vi "四通道数据采集.vi"() -> ()   [LabVIEW 2012, in "Mlistbox Tools.lvlib"]
uses:
  Mlistbox Tools.lvlib
  ListBox/Custom Type/Read and Write Mode.ctl
  Method/Clear.vi
  Property/Set and Get Row or Col Head Strings.vi
  Method/Add Item.vi
  Method/Add Item Buffered.vi
  Method/Sort.vi
  ListBox/Listbox Tool.lvlib
panel:
  out "Selected Item":string[](array[string])
  in  "清除项目":bool
  in  "缓冲添加项目":bool
  in  "停止按钮":bool
  in  "多列列表框":i32(listbox)
  # "双击列首自动排序"
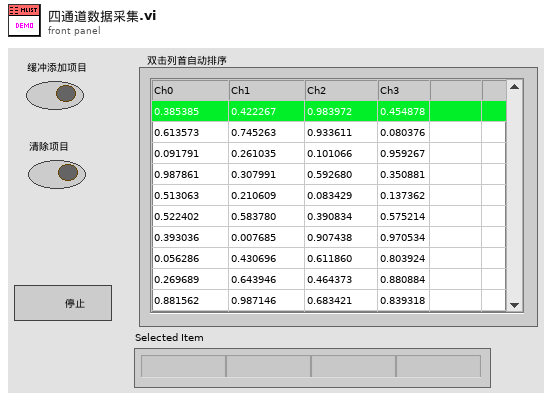
[diagram p1: front panel]
types:
  T1 = typedef "Listbox Tool.lvlib/Read and Write Mode.ctl" = enum16{"Read", "Write"}
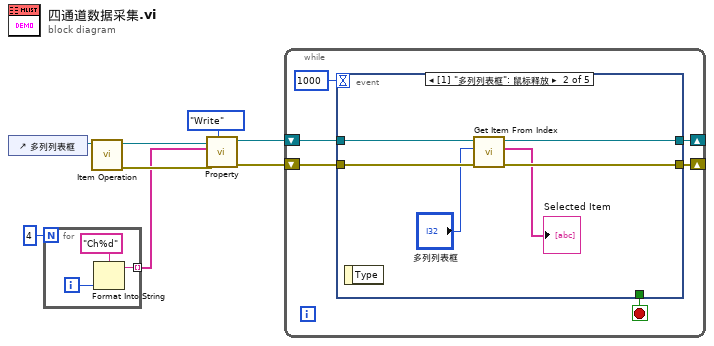
[diagram p0: block diagram]
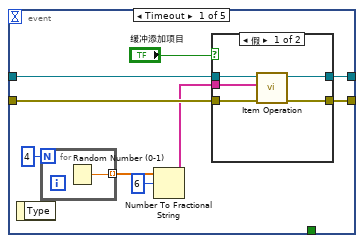
[diagram p2: hidden frame]
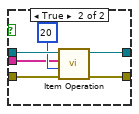
[diagram p3: hidden frame]
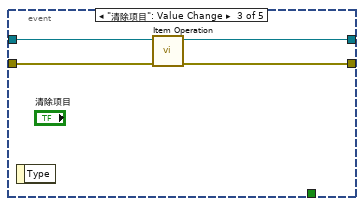
[diagram p4: hidden frame]
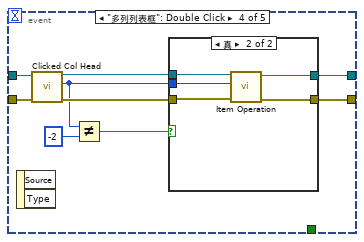
[diagram p5: hidden frame]
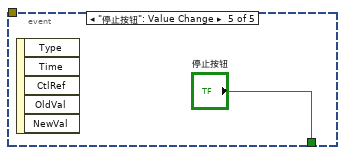
[diagram p7: hidden frame]
diagram:
  n1 = control-ref of="多列列表框"() -> (w8:refnum<vi>)
  n2 = for {
    N: 4 -> [_]
    tunnel: [w9] -> w4 mode=indexing
    i -> [w11]
    n3 = Format Into String(format string="Ch%d" ("格式字符串"), w11) -> (resulting string=w9:string)  [unwired: 2 in, 1 out]
  }
  n4 = call-poly "Item Operation.vi"("Mlistbox Ref"=w8) -> ("错误输出"=w6:errorcluster, "Mlistbox Ref Dup"=w7:refnum<vi>)  [unwired: 9 in]
  n5 = call-poly "Property.vi"("Mode"=Read_and_Write_Mode."Write", "错误输入"=w6, "String[]  In"=w4, "Mlistbox Ref"=w7) -> ("错误输出"=w1:errorcluster, "Mlistbox Ref Dup"=w2:refnum<vi>)  [unwired: 5 in, 1 out]
  n6 = while {
    shift-right: [w14] -> _
    shift-left: w2 -> [w15]
    shift-right: [w13] -> _
    shift-left: w1 -> [w16]
    stop <- w17 stop-if-true
    n7 = event shown="[1] \"多列列表框\": 鼠标释放" {
      selector: _ -> [_ _ _ _ _]
      dyn-events: _ -> [_ _ _ _ _]
      timeout: 1000 -> [_ _ _ _ _]
      tunnel: [_ _ _ _ "停止按钮"] -> w17
      tunnel: w16 -> [w26 w43 w47 w55 _]
      tunnel: w15 -> [w25 w44 w48 w54 _]
      tunnel: [w24 w41 w45 w57 _] -> w14
      tunnel: [w23 w42 w46 w56 _] -> w13
      event Timeout {
        n8 = event-data() -> ()  [unwired: 1 in, 1 out]
        n9 = for {
          N: 4 -> [_]
          tunnel: [w38] -> w21 mode=indexing
          n10 = Random Number (0-1)() -> (number: 0 to 1=w38:dbl)
        }
        n11 = Number To Fractional String(number=w21, width (-)=i16 6 ("宽度(-)")) -> (F-format string=w20:string[])  [unwired: 2 in]
        n12 = case shown="假" "缓冲添加项目" {
          tunnel: w26 -> [w31 w37]
          tunnel: w25 -> [w28 w36]
          tunnel: [w29 w35] -> w24
          tunnel: [w30 w34] -> w23
          tunnel: w20 -> [w27 w32]
          frame False {
            n13 = call-poly "Item Operation.vi"("错误输入"=w31, "Item"=w27, "Mlistbox Ref"=w28) -> ("错误输出"=w30:errorcluster, "Mlistbox Ref Dup"=w29:refnum<vi>)  [unwired: 7 in]
          }
          frame True {
            n14 = call-poly "Item Operation.vi"("错误输入"=w37, "Length"=20, "Item"=w32, "Mlistbox Ref"=w36) -> ("错误输出"=w34:errorcluster, "Mlistbox Ref Dup"=w35:refnum<vi>)  [unwired: 6 in]
          }
        }
      }
      event "多列列表框": Mouse Up {
        n15 = event-data() -> ()  [unwired: 1 in, 1 out]
        n16 = call "Get Item From Index.vi"("错误输入"=w43, "Index"="多列列表框", "Mlistbox Ref"=w44) -> ("错误输出"=w42:errorcluster, "Item"=→"Selected Item":string[], "Mlistbox Ref Dup"=w41:refnum<vi>)  [unwired: 6 in]
      }
      event "清除项目": Value Change {
        n17 = event-data() -> ()  [unwired: 1 in, 1 out]
        n18 = call-poly "Item Operation.vi"("错误输入"=w47, "Mlistbox Ref"=w48) -> ("错误输出"=w46:errorcluster, "Mlistbox Ref Dup"=w45:refnum<vi>)  [unwired: 8 in]
      }
      event "多列列表框": Double Click {
        n19 = event-data() -> ()  [unwired: 1 in, 2 out]
        n20 = call "Clicked Col Head.vi"("错误输入（无错误）"=w55, "Ref"=w54) -> ("错误输出"=w52:errorcluster, "Clicked Col Head"=w49:i32, "Dup Ref"=w53:refnum<vi>)  [unwired: 7 in]
        n21 = Not Equal?(x=w49, y=-2) -> (x != y?=w50:bool)
        n22 = case shown="真" w50 {
          tunnel: w53 -> [w59 w62]
          tunnel: w52 -> [w58 w61]
          tunnel: [w59 w64] -> w57
          tunnel: [w58 w63] -> w56
          tunnel: w49 -> [_ w60]
          frame False {
          }
          frame True {
            n23 = call-poly "Item Operation.vi"("错误输入"=w61, "列索引"=w60, "Mlistbox Ref"=w62) -> ("错误输出"=w63:errorcluster, "Mlistbox Ref Dup"=w64:refnum<vi>)  [unwired: 7 in]
          }
        }
      }
      event "停止按钮": Value Change {
        n24 = event-data() -> ()  [unwired: 1 in, 5 out]
      }
    }
  }
